vi "Format Str.vi"(8 "error in (no error)":errorcluster, 10 "Input Cmd String":string, 11 "VISA resource name":refnum<visa-resource-name>) -> (0 "error out":errorcluster, 2 "Formatted Cmd String":string, 3 "VISA resource name out":refnum<visa-resource-name>)   [LabVIEW 2018, in "EFD Ultimus V.lvlib"]
doc: "This VI will take the input command, determine the length of the command, compute the checksum, and concatenate the string to the correct command format. For example input Cmd String = UD-- where -- is space space. Formatted Cmd String= STX04UD C3ETX"
uses:
  EFD Ultimus V.lvlib
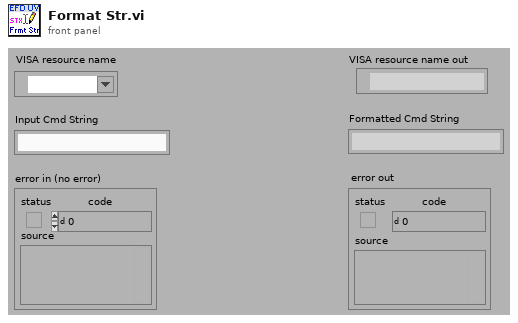
[diagram p1: front panel]
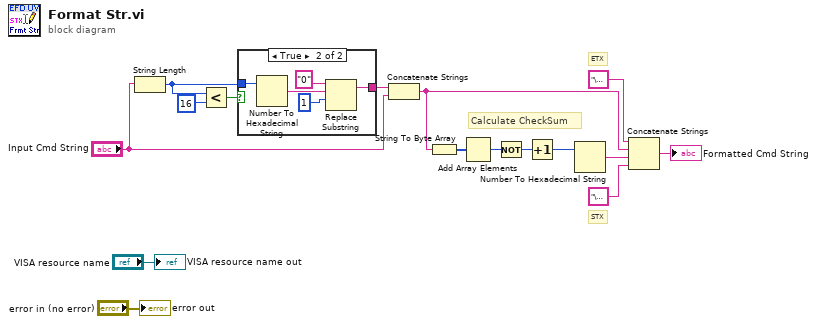
[diagram p0: block diagram]
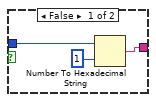
[diagram p2: hidden frame]
diagram:
  # "Calculate CheckSum"
  # "ETX"
  # "STX"
  n1 = String Length(string="Input Cmd String") -> (length=w15:i32)
  n2 = Less?(x=w15, y=16) -> (x < y?=w14:bool)
  n3 = case shown="True" w14 {
    tunnel: w15 -> [w19 w21]
    tunnel: [w17 w20] -> w16
    frame False {
      n4 = Number To Hexadecimal String(1:i16 1 ("width (-)"), 2:w19) -> (0:w17:string)
    }
    frame True {
      n5 = Number To Hexadecimal String(2:w21) -> (0:w22:string)  [unwired: 1 out]
      n6 = Replace Substring(3:1 ("offset (0)"), 4:w22, 5:"0" ("string")) -> (1:w20:string)  [unwired: 2 out]
    }
  }
  n7 = Concatenate Strings(w16, "Input Cmd String") -> (w4:string)
  n8 = String To Byte Array(string=w4) -> (unsigned byte array=w8:u8[])
  n9 = Add Array Elements(numeric array=w8) -> (sum=w5:u8)
  n10 = Not(x=w5) -> (.not. x?=w6:u8)
  n11 = Increment(x=w6) -> (x+1=w7:u8)
  n12 = Number To Hexadecimal String(2:w7) -> (0:w3:string)  [unwired: 1 out]
  n13 = Concatenate Strings("\u0002" ("STX"), w4, w3, "\u0003" ("string")) -> (→"Formatted Cmd String":string)
  "error out" <- "error in (no error)"
  "VISA resource name out" <- "VISA resource name"
